vi "Page_Source_Settings_Initialize.vi"(8 "error in (no error)":errorcluster, 9 "ctlReferences":T1, 11 "AB_DLL in":refnum<class "AB_DLL.lvclass">) -> (0 "error out":errorcluster, 1 "supportedFunctions":T2, 3 "AB_DLL out":refnum<class "AB_DLL.lvclass">)   [LabVIEW 2020, in "AB_DLL.lvclass"]
uses:
  <vilib>/AppBuilder/AB_Classes/DLL/AB_DLL.lvclass
  <resource>/Framework/Providers/Builds/AppBuilder/AB_UI_Page_Source_Settings_supportedFunctions.ctl
  <resource>/Framework/Providers/Builds/AppBuilder/AB_UI_Page_Source_Settings_References.ctl
  <resource>/Framework/Providers/Common/provcom_StringGlobals.vi
  <vilib>/AppBuilder/AB_Classes/Application/AB_Application.lvclass
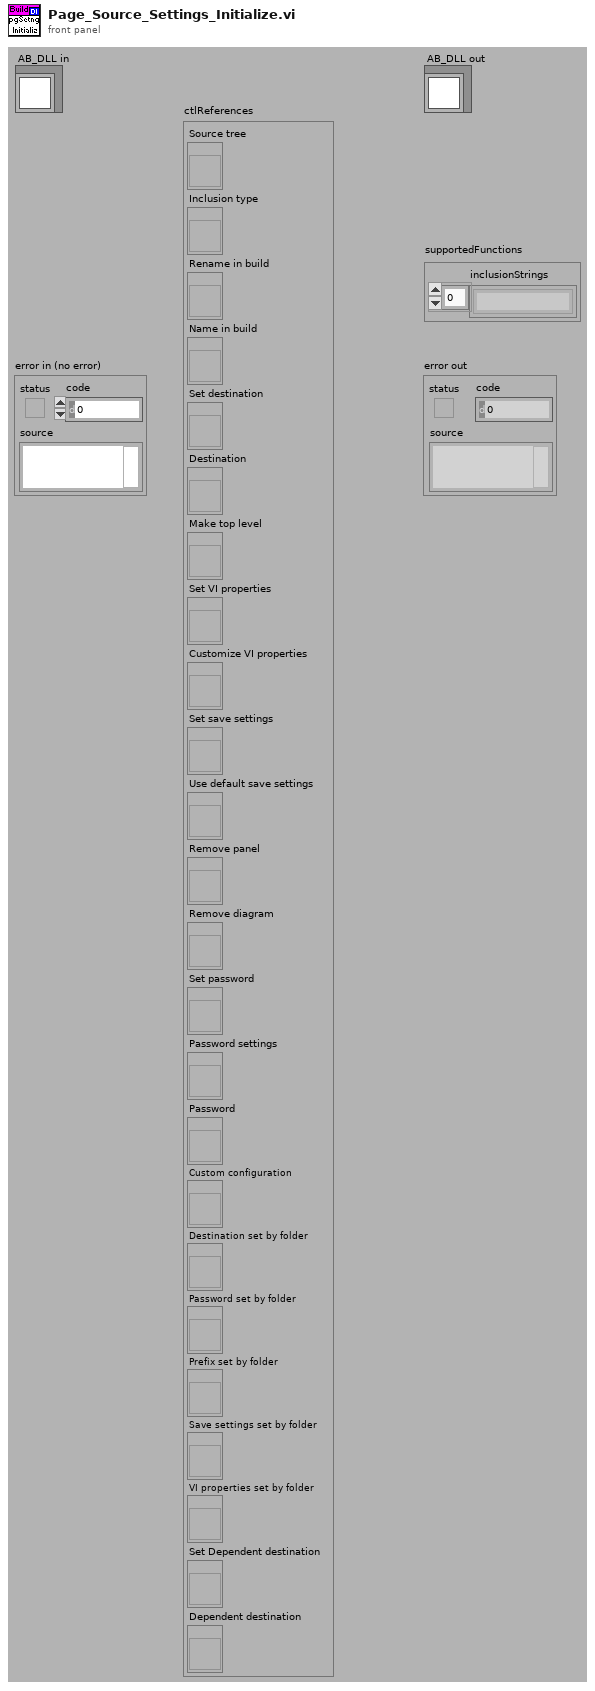
[diagram p1: front panel]
types:
  T1 = typedef "AB_UI_Page_Source_Settings_References.ctl" = cluster{"Source tree":refnum<vi>, "Inclusion type":refnum<vi>, "Rename in build":refnum<vi>, "Name in build":refnum<vi>, "Set destination":refnum<vi>, "Destination":refnum<vi>, "Make top level":refnum<vi>, "Set VI properties":refnum<vi>, "Customize VI properties":refnum<vi>, "Set save settings":refnum<vi>, "Use default save settings":refnum<vi>, "Remove panel":refnum<vi>, "Remove diagram":refnum<vi>, "Set password":refnum<vi>, "Password settings":refnum<vi>, "Password":refnum<vi>, "Custom configuration":refnum<vi>, "Destination set by folder":refnum<vi>, "Password set by folder":refnum<vi>, "Prefix set by folder":refnum<vi>, "Save settings set by folder":refnum<vi>, "VI properties set by folder":refnum<vi>, "Set Dependent destination":refnum<vi>, "Dependent destination":refnum<vi>}
  T2 = typedef "AB_UI_Page_Source_Settings_supportedFunctions.ctl" = cluster{"inclusionStrings":string[]}
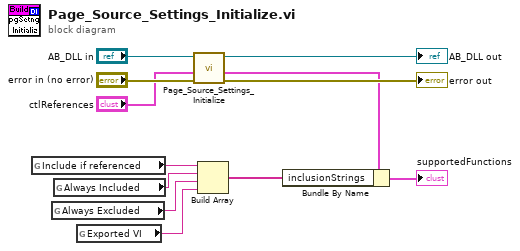
[diagram p0: block diagram]
diagram:
  n1 = global read "provcom_StringGlobals.vi" "Include if referenced"() -> (w3:string)
  n2 = global read "provcom_StringGlobals.vi" "Always Excluded"() -> (w5:string)
  n3 = global read "provcom_StringGlobals.vi" "Always Included"() -> (w4:string)
  n4 = global read "provcom_StringGlobals.vi" "Exported VI"() -> (w2:string)
  n5 = call-parent "Page_Source_Settings_Initialize.vi"("error in (no error)"="error in (no error)", "ctlReferences"="ctlReferences", "AB_Build in"="AB_DLL in") -> ("error out"=→"error out":errorcluster, "supportedFunctions"=w7:T2, "AB_Build out"=→"AB_DLL out":refnum<class "AB_DLL.lvclass">)  [unwired: 6 in]
  n6 = Build Array(w3, w4, w5, w2) -> (w1:string[])
  n7 = Bundle By Name(cluster=w7, "inclusionStrings"=w1) -> (→"supportedFunctions":T2)
